vi "Waveform Attribute, Get DBL Reference.vi"(5 "DigNum Refnum":refnum<vi>, 6 "error in":errorcluster, 9 "waveform":waveform(dbl)) -> (0 "error out":errorcluster, 1 "new value":dbl=nan format="%.3f", 2 "Label.Text":string, 3 "waveform dup":waveform(dbl)={"t0"=timestamp(0 s since 1904-01-01), "dt"=nan, "Y"=[]}, 4 "found":bool)   [LabVIEW 2010]
doc: "Reads a numeric value from a waveform attribute using a control reference."
panel:
  out "old value":dbl=nan format="%.3f"
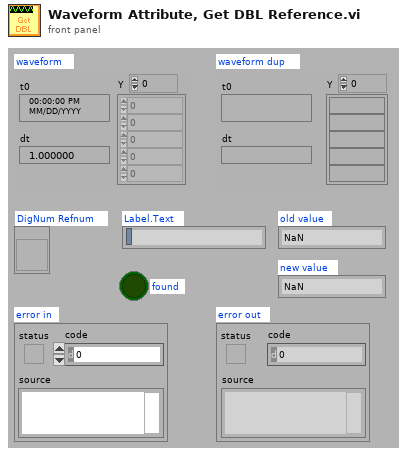
[diagram p1: front panel]
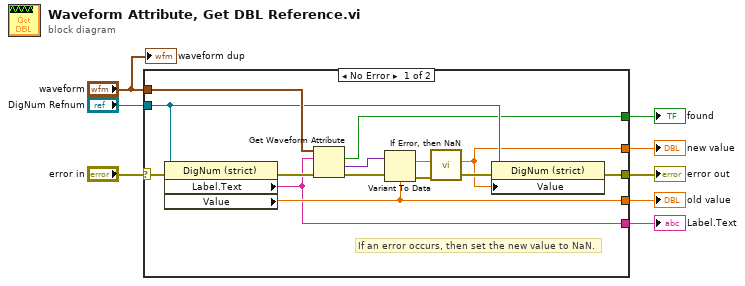
[diagram p0: block diagram]
diagram:
  n1 = case shown="No Error" "error in" {
    selector: "error in" -> [w20 w23]
    tunnel: "DigNum Refnum" -> [w18 _]
    tunnel: [w19 w23] -> w7
    tunnel: "waveform" -> [w21 _]
    tunnel: [w17 _] -> w5
    tunnel: [w15 _] -> w3
    tunnel: [w9 _] -> w2
    tunnel: [w14 _] -> w1
    frame No Error {
      # "If an error occurs, then set the new value to NaN."
      n2 = property class="DigNum (strict)"(reference=w18, error in=w20) -> (error out=w22:errorcluster, "Label.Text"=w14:string, "Value"=w15:dbl)  [unwired: 1 out]
      n3 = Get Waveform Attribute(4:w22, 6:w14, 7:w21) -> (0:w13:errorcluster, 1:w16:variant, 2:w17:bool)  [unwired: 1 in, 1 out]
      n4 = Variant To Data(error in=w13, Variant=w16, type=w15) -> (error out=w11:errorcluster, data=w10:dbl)
      n5 = call "If Error, then NaN.vi"("error in (T)"=w11, "value2"=w10) -> ("error out"=w12:errorcluster, "value out2"=w9:dbl)  [unwired: 4 in, 2 out]
      n6 = property class="DigNum (strict)"(reference=w18, error in=w12, "Value"=w9) -> (error out=w19:errorcluster)  [unwired: 1 out]
    }
    frame Error {
    }
  }
  "error out" <- w7
  "found" <- w5
  "old value" <- w3
  "new value" <- w2
  "Label.Text" <- w1
  "waveform dup" <- "waveform"
